vi "CreateFile (SubVI).vi"(0 "Path name":path, 5 "Save Data":bool, 7 "File name":string, 9 "Date Folder":bool, 11 "error in (no error)":errorcluster, 12 "Add time to file name":bool) -> (4 "Byte Stream File out":refnum<file>, 6 "String":string, 15 "error out":errorcluster)   [LabVIEW 2021]
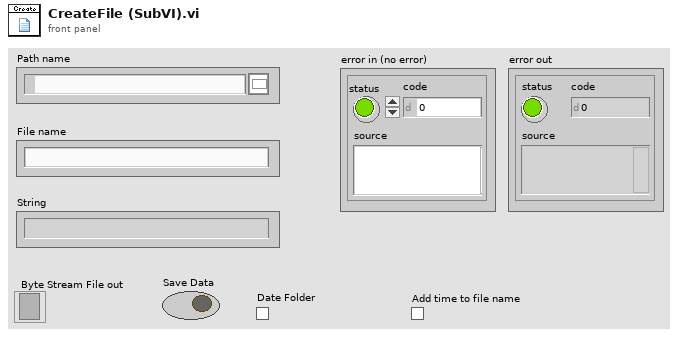
[diagram p1: front panel]
types:
  T1 = enum16{"open", "replace", "create", "open or create", "replace or create", "replace or create with confirmation"}
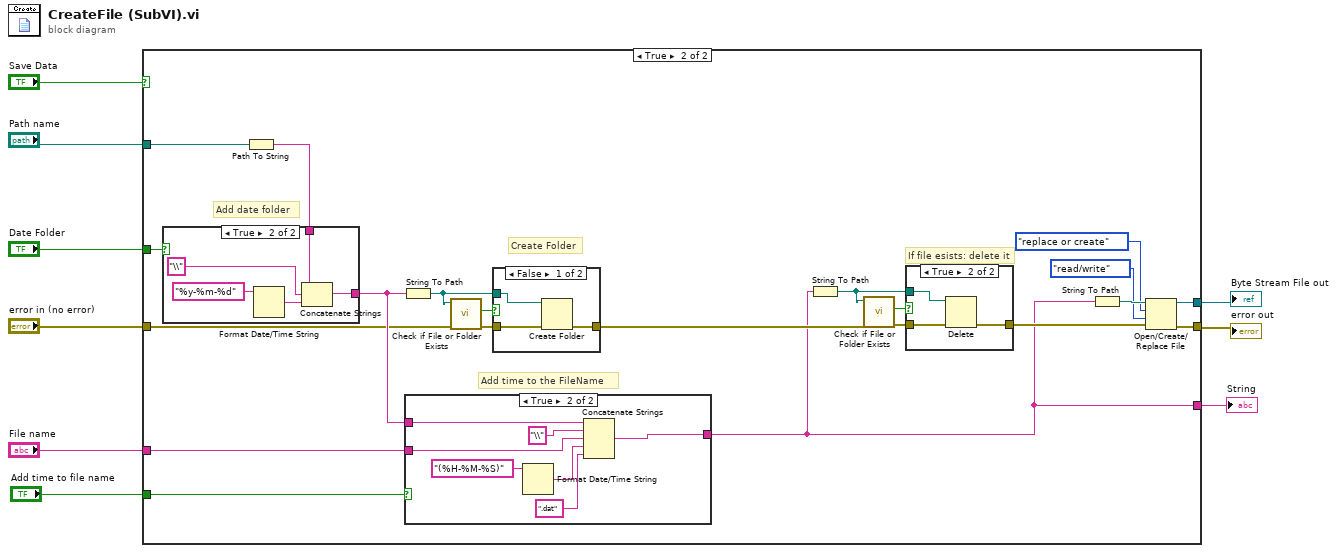
[diagram p0: block diagram]
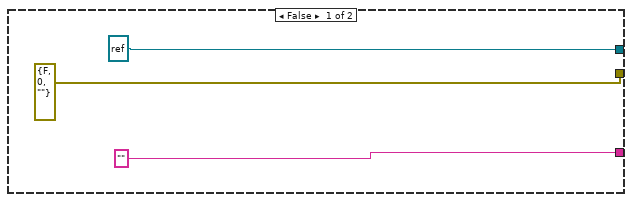
[diagram p2: hidden frame]
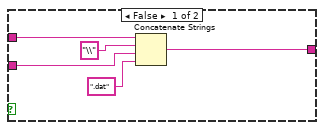
[diagram p3: hidden frame]
diagram:
  n1 = case shown="True" "Save Data" {
    tunnel: [refnum<file> refnum ("refnum out") w33] -> w4
    tunnel: [errorcluster {"status"=FALSE, "code"=0, "source"=""} ("error out") w32] -> w5
    tunnel: "Path name" -> [_ w28]
    tunnel: "File name" -> [_ w25]
    tunnel: ["" w14] -> w9
    tunnel: "error in (no error)" -> [_ w23]
    tunnel: "Date Folder" -> [_ w20]
    tunnel: "Add time to file name" -> [_ w13]
    frame False {
    }
    frame True {
      # "Add time to the FileName"
      # "Add date folder"
      # "If file esists: delete it"
      # "Create Folder"
      n2 = Path To String(path=w28) -> (string=w29:string)
      n3 = case shown="True" w20 {
        tunnel: w29 -> [w50 w52]
        tunnel: [w50 w51] -> w26
        frame False {
        }
        frame True {
          n4 = Format Date/Time String(time format string (%c)="%y-%m-%d") -> (date/time string=w54:string)  [unwired: 2 out]
          n5 = Concatenate Strings(w52, "\\" ("string"), w54) -> (w51:string)
        }
      }
      n6 = String To Path(string=w26) -> (path=w27:path)
      n7 = case shown="True" w13 {
        tunnel: w26 -> [w38 w45]
        tunnel: w25 -> [w36 w43]
        tunnel: [w34 w42] -> w14
        frame False {
          n8 = Concatenate Strings(w38, "\\" ("string"), w36, ".dat" ("string")) -> (w34:string)
        }
        frame True {
          n9 = Format Date/Time String(time format string (%c)="(%H-%M-%S)") -> (date/time string=w39:string)  [unwired: 2 out]
          n10 = Concatenate Strings(w45, "\\" ("string"), w43, w39, ".dat" ("string")) -> (w42:string)
        }
      }
      n11 = call <vilib>:"Check if File or Folder Exists.vi"("error in (no error)"=w23, "path"=w27) -> ("error out"=w30:errorcluster, "file or folder exists?"=w31:bool)  [unwired: 7 in, 1 out]
      n12 = case shown="False" w31 {
        tunnel: w30 -> [w58 w59]
        tunnel: [w57 w59] -> w15
        tunnel: w27 -> [w56 _]
        frame False {
          n13 = Create Folder(path (use dialog)=w56, error in=w58) -> (error out=w57:errorcluster)  [unwired: 1 in, 2 out]
        }
        frame True {
        }
      }
      n14 = String To Path(string=w14) -> (path=w17:path)
      n15 = call <vilib>:"Check if File or Folder Exists.vi"("error in (no error)"=w15, "path"=w17) -> ("error out"=w18:errorcluster, "file or folder exists?"=w19:bool)  [unwired: 7 in, 1 out]
      n16 = case shown="True" w19 {
        tunnel: w18 -> [w46 w48]
        tunnel: [w46 w47] -> w16
        tunnel: w17 -> [_ w49]
        frame False {
        }
        frame True {
          n17 = Delete(path (use dialog)=w49, error in=w48) -> (error out=w47:errorcluster)  [unwired: 3 in, 2 out]
        }
      }
      n18 = String To Path(string=w14) -> (path=w24:path)
      n19 = Open/Create/Replace File(file path (use dialog)=w24, error in=w16, operation (0:open)=T1."replace or create", access (0:read/write)=enum16{"read/write", "read-only", "write-only"}."read/write") -> (refnum out=w33:refnum<file>, error out=w32:errorcluster)  [unwired: 2 in, 1 out]
    }
  }
  "String" <- w9
  "error out" <- w5
  "Byte Stream File out" <- w4
